vi "Xbox One Controller - Find Controllers.vi"() -> ()   [LabVIEW 2011, in "LMH-Xbox-One-Controller.lvlib"]
doc: "This example demonstrates how find the device index of all available Xbox One controllers."
uses:
  vi.lib/MakerHub/Xbox-One-Controller/LMH-Xbox-One-Controller.lvlib
  vi.lib/MakerHub/Xbox-One-Controller/Private/Type Defs/Xbox Controller Device.ctl
panel:
  out "Xbox Controllers":T1[](array[typedef])
  # "Xbox One Controller - Find Controllers\n\nThis example demonstrates how find the index associated with an Xbox One Controller.\n\nInstructions\n1. Click the Run Arrow.\n2. Notice the controller data indicator updates with all Xbox One Controller indexes."
  # "Controller Data"
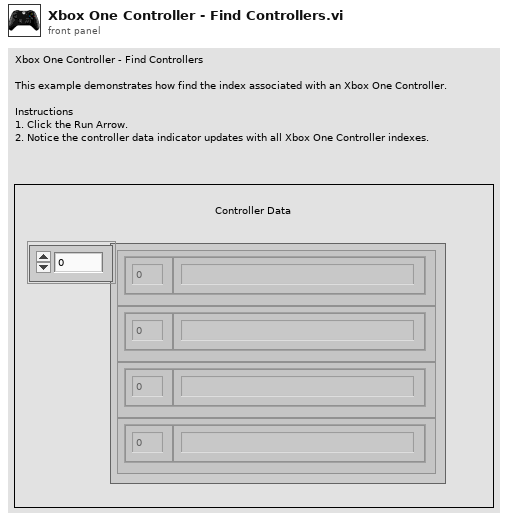
[diagram p1: front panel]
types:
  T1 = typedef "LMH-Xbox-One-Controller.lvlib/Xbox Controller Device.ctl" = cluster{"Device Index":i32, "Device Name":string}
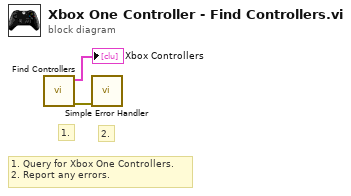
[diagram p0: block diagram]
diagram:
  # "1. Query for Xbox One Controllers.\n2. Report any errors."
  # "2."
  # "1."
  n1 = call "Find Controllers.vi"() -> ("Error Out"=w2:errorcluster, "Xbox Controllers"=→"Xbox Controllers":T1[])  [unwired: 10 in]
  n2 = call <vilib>:"Simple Error Handler.vi"("error in (no error)"=w2) -> ()  [unwired: 4 in, 5 out]
